vi "SVL Running RMS Level.vi"   [LabVIEW 2017, in "SoundVib_VibrationLevel.lvlib"]
doc: "Computes the running root-mean-square (RMS) level of <B>scaled signal [EU]</B> or <B>even-angle signal [EU]</B>. <B>scaled signal [EU]</B> should have a zero DC component. You can attenuate the DC component with hardware AC-coupling filters and with software high-pass filters. <B>integration time [s]</B> and <B>integration revolutions</B> specify the duration over which the RMS level is computed. A new running RMS value is returned each time you call this VI. A shift register internal to this VI maintains the result of past runs. The new result is an averaged level that includes the latest block of samples and the level history in the specified integration time. Wire data to the <B>scaled signal [EU]</B> input to determine the polymorphic instance to use or manually select the instance."
uses:
  <vilib>/addons/Sound and Vibration/svt_Level/SoundVib_VibrationLevel.lvlib
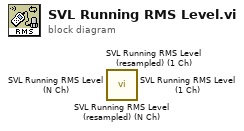
[diagram p0: block diagram]
diagram:
  n1 = call <vilib>:"SVL Running RMS Level (resampled) (N Ch).vi"() -> ()  [unwired: 8 in, 4 out]
  n2 = call <vilib>:"SVL Running RMS Level (resampled) (1 Ch).vi"() -> ()  [unwired: 8 in, 4 out]
  n3 = call <vilib>:"SVL Running RMS Level (N Ch).vi"() -> ()  [unwired: 8 in, 4 out]
  n4 = call <vilib>:"SVL Running RMS Level (1 Ch).vi"() -> ()  [unwired: 8 in, 4 out]
